vi "HSDIO_6541_Check_Wfm_Existence.vi"(8 "error  in":errorcluster caption="error in", 9 "TIMING Inputs":T2={"Number of Acquisitions "=1, "Number of Accumulations"=1, "Table of Waveforms"=[], "Script Text"=""} {"Number of Accumulations" min=0 max=50 step=1; "Number of Acquisitions" min=1 max=10 step=1}, 10 "SOFTWARE Inputs":T1={"Application Directory"=path "D:/S.O.F.T.S/LABVIEW/PIL", "Software Version"="1.0.0", "Data Path"=path "D:/PIRENEA/DATA", "XML Path"=path "D:/PIRENEA/DATA", "XML File Filter"="*.xml", "XML Saved Path"=path "D:/PIRENEA/DATA/SAVED", "Excit Scripts Path"=path "D:/PIRENEA/TECHNICAL/EXCIT_SCRIPTS", "Excit Scripts File Filter"="*.txt", "Excit Waveforms Path"=path "D:/PIRENEA/TECHNICAL/EXCIT_WFMS", "Excit Waveforms File Filter"="*.bin", "Timing Scripts Path"=path "D:/PIRENEA/TECHNICAL/TIMING_SCRIPTS", "Timing Scripts File Filter"="*.txt", "Timing Waveforms Path"=path "D:/PIRENEA/TECHNICAL/TIMING_WFMS", "Timing Waveforms File Filter"="*.bin", "Trapping Waveforms Path"=path "D:/PIRENEA/TECHNICAL/TRAPPING_WFMS", "Trapping Waveforms File Filter"="*.bin"}) -> (0 "error out":errorcluster)   [LabVIEW 2017]
doc: "This VI checks if the timing waveforms required by the script are present on disk.\n\n1. The path ofr waveforms and script has to be checked before running this VI.\n2. If a waveform is missing, this VI generates an error message."
uses:
  controls/TIMING_Inputs.ctl
  controls/SOFTWARE_Inputs.ctl
  <vilib>/Utility/error.llb/Error Cluster From Error Code.vi
  <vilib>/ErrorRing/Error Ring.xnode
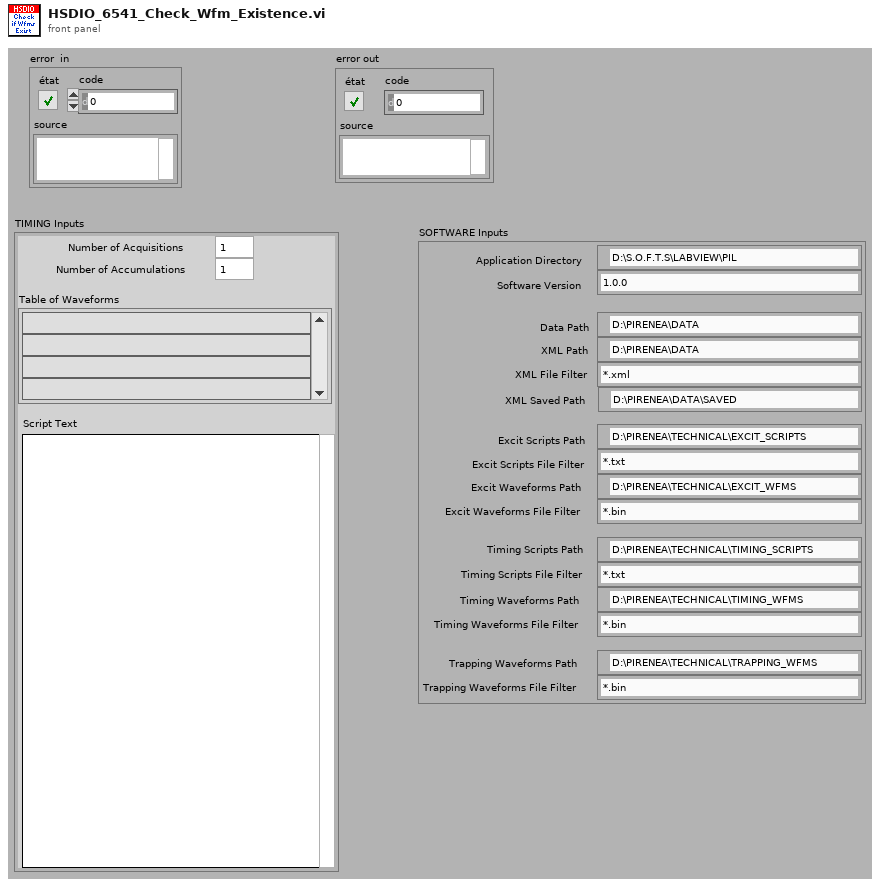
[diagram p1: front panel]
types:
  T1 = typedef "SOFTWARE_Inputs.ctl" = cluster{"Application Directory":path, "Software Version":string, "Data Path":path, "XML Path":path, "XML File Filter":string, "XML Saved Path":path, "Excit Scripts Path":path, "Excit Scripts File Filter":string, "Excit Waveforms Path":path, "Excit Waveforms File Filter":string, "Timing Scripts Path":path, "Timing Scripts File Filter":string, "Timing Waveforms Path":path, "Timing Waveforms File Filter":string, "Trapping Waveforms Path":path, "Trapping Waveforms File Filter":string}
  T2 = typedef "TIMING_Inputs.ctl" = cluster{"Number of Acquisitions ":i16, "Number of Accumulations":i16, "Table of Waveforms":string[], "Script Text":string}
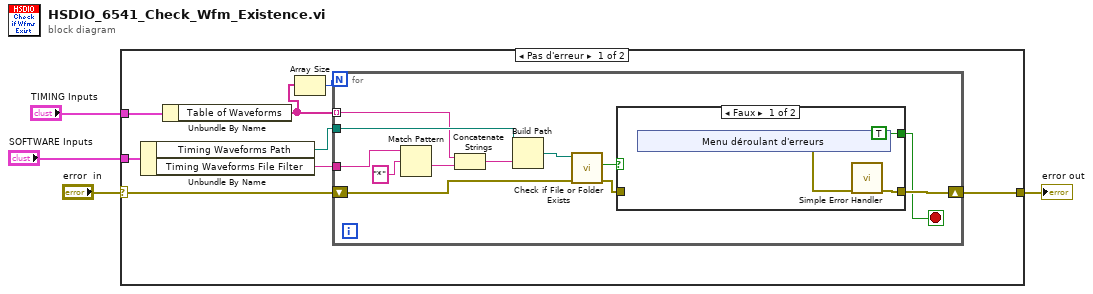
[diagram p0: block diagram]
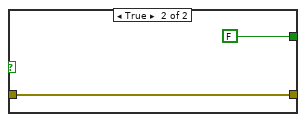
[diagram p2: hidden frame]
diagram:
  n1 = case shown="Pas d'erreur" "error  in" {
    selector: "error  in" -> [w12 w35]
    tunnel: [w7 w35] -> w4
    tunnel: "SOFTWARE Inputs" -> [w11 _]
    tunnel: "TIMING Inputs" -> [w8 _]
    frame No Error {
      n2 = Unbundle By Name(w11) -> ("Timing Waveforms Path"=w10:path, "Timing Waveforms File Filter"=w9:string)
      n3 = Unbundle By Name(w8) -> ("Table of Waveforms"=w6:string[])
      n4 = Array Size(array=w6) -> (size(s)=w5:i32)
      n5 = for {
        N: w5 -> [_]
        tunnel: w6 -> [w20] mode=indexing
        tunnel: w10 -> [w24]
        tunnel: w9 -> [w23]
        shift-right: [w15] -> w7
        shift-left: w12 -> [w17]
        stop <- w13 stop-if-true
        n6 = Match Pattern(string=w23, regular expression="*" ("expression régulière")) -> (after substring=w21:string)  [unwired: 1 in, 3 out]
        n7 = Concatenate Strings(w20, w21) -> (w14:string)
        n8 = Build Path(base path=w24, name or relative path=w14) -> (appended path=w19:path)
        n9 = call <vilib>:"Check if File or Folder Exists.vi"("error in (no error)"=w17, "path"=w19) -> ("error out"=w16:errorcluster, "file or folder exists?"=w18:bool)  [unwired: 7 in, 1 out]
        n10 = case shown="Faux" w18 {
          tunnel: [w27 w34] -> w15
          tunnel: w16 -> [_ w34]
          tunnel: [TRUE FALSE] -> w13
          frame False {
            n11 = xnode "Menu déroulant d'erreurs"() -> ("sortie d'erreur"=w26:errorcluster)
            n12 = call <vilib>:"Simple Error Handler.vi"("error in (no error)"=w26) -> ("error out"=w27:errorcluster)  [unwired: 4 in, 4 out]
          }
          frame True {
          }
        }
      }
    }
    frame Error {
    }
  }
  "error out" <- w4
